vi "SetShutterModes.vi"(8 "Error In":errorcluster, 10 "Shutters":T1, 11 "Operational Mode":T4) -> (0 "Error Out":errorcluster, 2 "Shutters out":T1)   [LabVIEW 2016]
uses:
  Controls/Operational Modes.ctl
  Controls/Shutters.ctl
  Controls/Shutter Data.ctl
  Controls/Shutter States.ctl
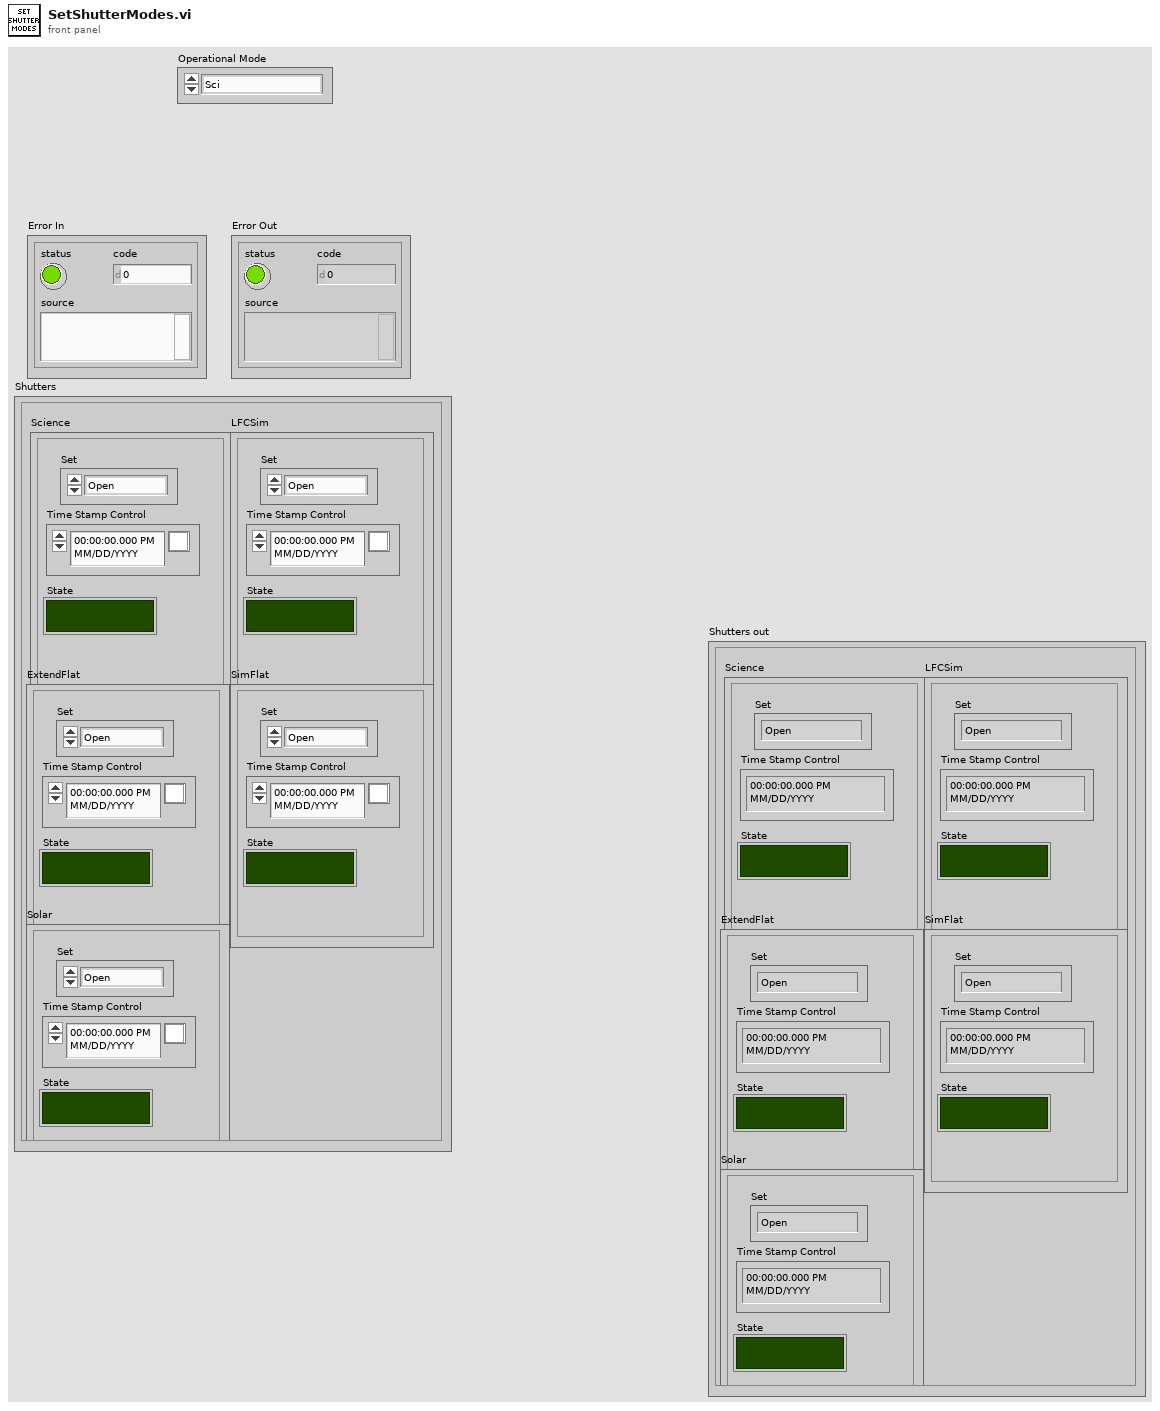
[diagram p1: front panel]
types:
  T1 = typedef "Shutters.ctl" = cluster{"Science":T2, "LFCSim":T2, "ExtendFlat":T2, "SimFlat":T2, "Solar":T2}
  T2 = typedef "Shutter Data.ctl" = cluster{"Time Stamp Control":timestamp, "State":bool, "Set":T3}
  T3 = typedef "Shutter States.ctl" = enum16{"Open", "Close", "Wait", "Off", "Arm", "Idle"}
  T4 = typedef "Operational Modes.ctl" = enum16{"Sci", "Sci-LFC", "Solar", "Solar-LFC", "LFC", "LFC-Sim", "LFC-Both", "ThAr", "ThAr-LFC", "Flat", "ExtFlat", "ExtFlat-Sim", "ExtFlat-Both", "Qtz", "ExtQtz", "ExtQtz-Sim", "ExtQtz-Both", "Dark", "Manual", "Off"}
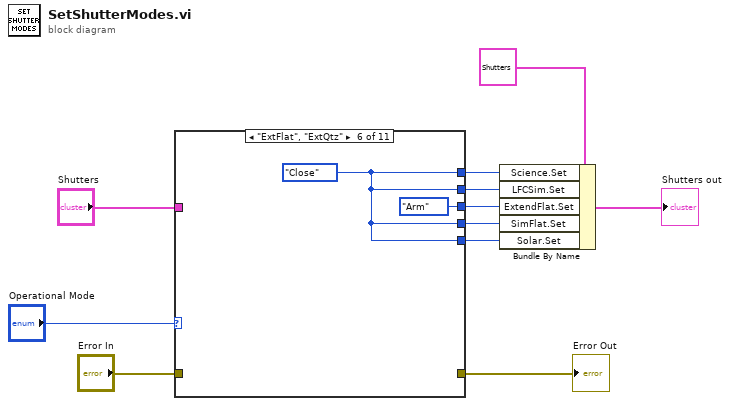
[diagram p0: block diagram]
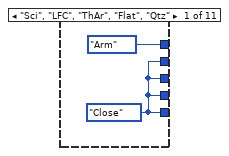
[diagram p2: hidden frame]
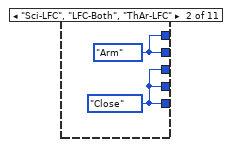
[diagram p3: hidden frame]
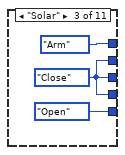
[diagram p4: hidden frame]
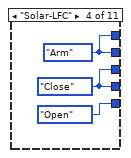
[diagram p5: hidden frame]
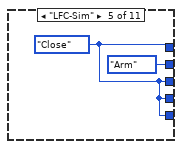
[diagram p6: hidden frame]
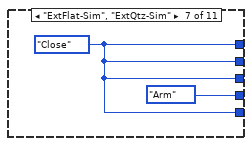
[diagram p7: hidden frame]
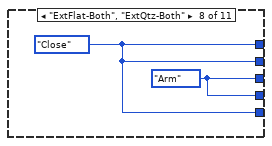
[diagram p8: hidden frame]
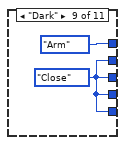
[diagram p9: hidden frame]
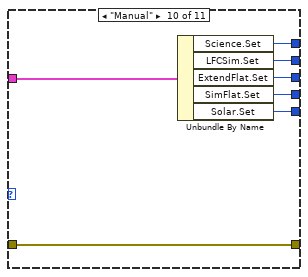
[diagram p10: hidden frame]
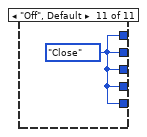
[diagram p11: hidden frame]
diagram:
  n1 = case shown="\"ExtFlat\", \"ExtQtz\"" "Operational Mode" {
    tunnel: [Shutter_States."Arm" ("Set") w15 Shutter_States."Arm" ("Set") w21 w22 w24 w26 w28 Shutter_States."Arm" ("Set") w33 w39] -> w11
    tunnel: [w12 w15 w17 w21 Shutter_States."Arm" ("Set") w24 w26 w28 w30 w34 w39] -> w7
    tunnel: [w12 w14 w17 w20 w22 Shutter_States."Arm" ("Set") w26 w29 w30 w35 w39] -> w10
    tunnel: [w12 w14 w17 w20 w22 w24 Shutter_States."Arm" ("Set") w29 w30 w36 w39] -> w9
    tunnel: [w12 w14 Shutter_States."Open" ("Set") Shutter_States."Open" ("Set") w22 w24 w26 w28 w30 w37 w39] -> w8
    tunnel: "Shutters" -> [_ _ _ _ _ _ _ _ _ w38 _]
    tunnel: "Error In" -> [_ _ _ _ _ _ _ _ _ w32 _]
    tunnel: [_ _ _ _ _ _ _ _ _ w32 _] -> w4
    frame "Sci", "LFC", "ThAr", "Flat", "Qtz" {
      w12 = Shutter_States."Close" ("Set")
    }
    frame "Sci-LFC", "LFC-Both", "ThAr-LFC" {
      w14 = Shutter_States."Close" ("Set")
      w15 = Shutter_States."Arm" ("Set")
    }
    frame "Solar" {
      w17 = Shutter_States."Close" ("Set")
    }
    frame "Solar-LFC" {
      w20 = Shutter_States."Close" ("Set")
      w21 = Shutter_States."Arm" ("Set")
    }
    frame "LFC-Sim" {
      w22 = Shutter_States."Close" ("Set")
    }
    frame "ExtFlat", "ExtQtz" {
      w24 = Shutter_States."Close" ("Set")
    }
    frame "ExtFlat-Sim", "ExtQtz-Sim" {
      w26 = Shutter_States."Close" ("Set")
    }
    frame "ExtFlat-Both", "ExtQtz-Both" {
      w28 = Shutter_States."Close" ("Set")
      w29 = Shutter_States."Arm" ("Set")
    }
    frame "Dark" {
      w30 = Shutter_States."Close" ("Set")
    }
    frame "Manual" {
      n2 = Unbundle By Name(w38) -> ("Science.Set"=w33:T3, "LFCSim.Set"=w34:T3, "ExtendFlat.Set"=w35:T3, "SimFlat.Set"=w36:T3, "Solar.Set"=w37:T3)
    }
    frame "Off", Default {
      w39 = Shutter_States."Close" ("Set")
    }
  }
  "Error Out" <- w4
  n3 = Bundle By Name(cluster=T1 {"Science"={"Time Stamp Control"=timestamp(0 s since 1904-01-01), "State"=FALSE, "Set"=enum."Open"}, "LFCSim"={"Time Stamp Control"=timestamp(0 s since 1904-01-01), "State"=FALSE, "Set"=enum."Open"}, "ExtendFlat"={"Time Stamp Control"=timestamp(0 s since 1904-01-01), "State"=FALSE, "Set"=enum."Open"}, "SimFlat"={"Time Stamp Control"=timestamp(0 s since 1904-01-01), "State"=FALSE, "Set"=enum."Open"}, "Solar"={"Time Stamp Control"=timestamp(0 s since 1904-01-01), "State"=FALSE, "Set"=enum."Open"}} ("Shutters"), "Science.Set"=w11, "LFCSim.Set"=w7, "ExtendFlat.Set"=w10, "SimFlat.Set"=w9, "Solar.Set"=w8) -> (→"Shutters out":T1)
